vi "ATF-Pump-DO_Element to Waveform.vi"(9 "t0":timestamp[](array[timestamp]), 10 "size":i32, 11 "deleted portion":i16[][](array[numeric])) -> (3 "Array out":waveform(dbl)[](array[waveform]))   [LabVIEW 2022 SP3]
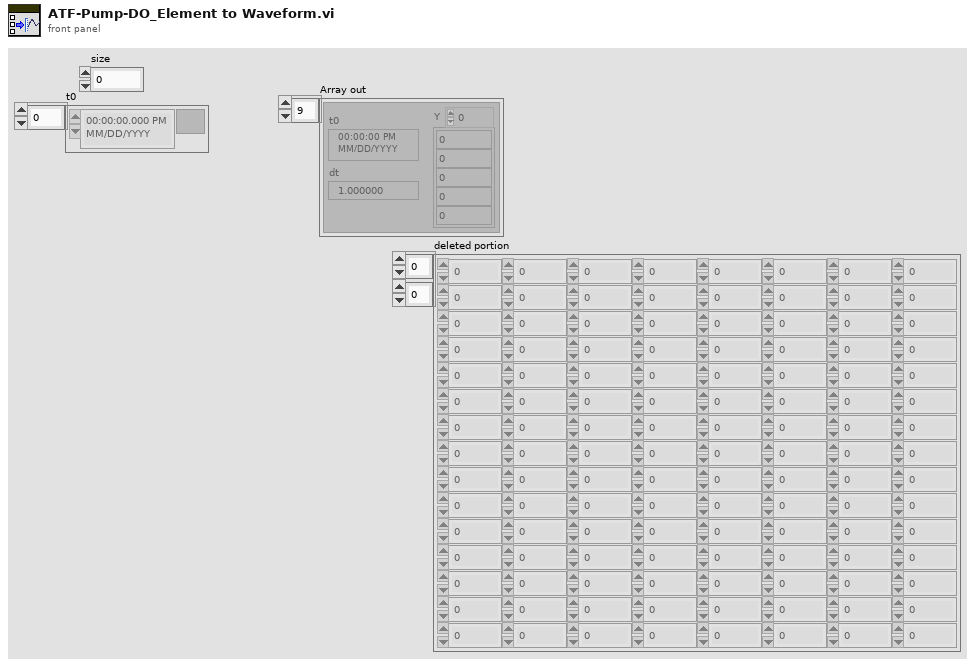
[diagram p1: front panel]
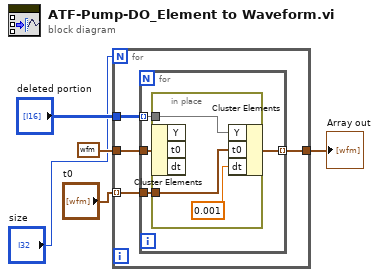
[diagram p0: block diagram]
diagram:
  n1 = for {
    N: "size" -> [_]
    tunnel: waveform(dbl) {"t0"=timestamp(0 s since 1904-01-01), "dt"=0.001, "Y"=[]} ("Waveform") -> [w9]
    tunnel: [w8] -> w4
    tunnel: "deleted portion" -> [w7]
    tunnel: "t0" -> [w6] mode=indexing
    n2 = for {
      tunnel: [w12] -> w8 mode=indexing
      tunnel: w9 -> [w13]
      tunnel: w7 -> [w11] mode=indexing
      tunnel: w6 -> [w10]
      n3 = in-place {
        in-place-border: w11 -> [w16]
        in-place-border: w10 -> [w15]
        n4 = in-place-cluster #1(w13) -> ()  [unwired: 3 out]
        n5 = in-place-cluster #1("Y"=w16, "t0"=w15, "dt"=0.001) -> (w12:waveform(dbl))
      }
    }
  }
  "Array out" <- w4
